vi "NI_9219_Config.vi"(8 "error in":errorcluster, 11 "task in":refnum<k21>) -> (0 "error out":errorcluster, 3 "task out":refnum<k21>)   [LabVIEW 2022 SP3]
uses:
  <vilib>/DAQmx/create/channels.llb/DAQmx Create Channel (AI-Voltage-Basic).vi
  <vilib>/DAQmx/create/channels.llb/DAQmx Create Channel (AI-Current-Basic).vi
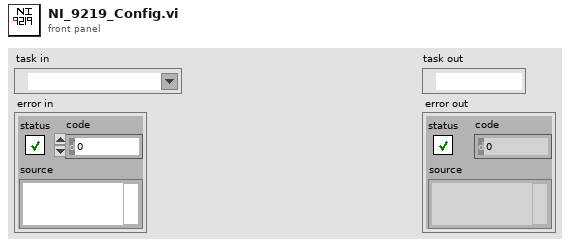
[diagram p1: front panel]
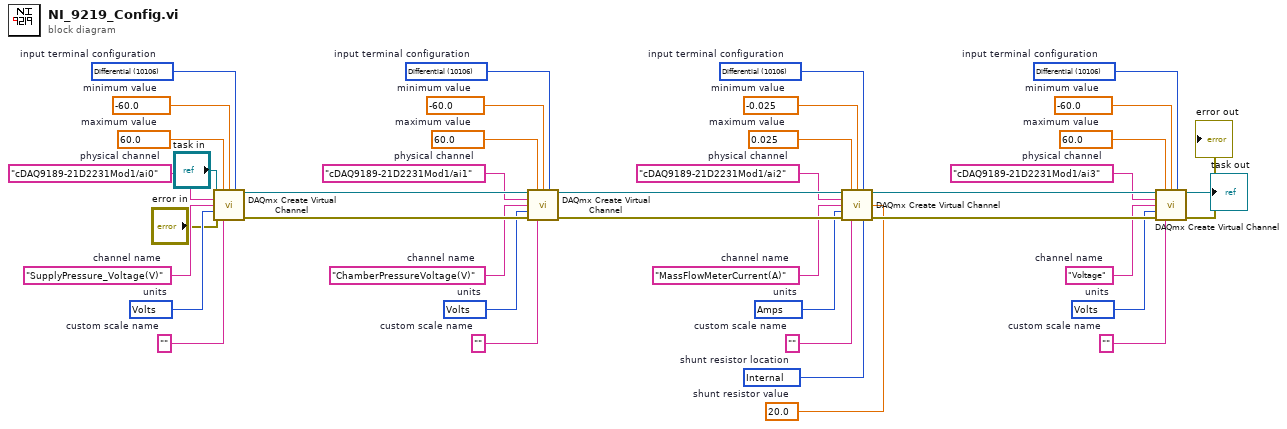
[diagram p0: block diagram]
diagram:
  w5 = 10106 items=["default"=-1, "RSE"=10083, "NRSE"=10078, "Differential"=10106, "Pseudodifferential"=12529]  # input terminal configuration
  w6 = 10348 items=["Volts"=10348, "From Custom Scale"=10065]  # units
  w7 = "Voltage"  # channel name
  w8 = ""  # custom scale name
  w9 = -60.0  # minimum value
  w10 = 60.0  # maximum value
  w11 = "cDAQ9189-21D2231Mod1/ai3"  # physical channel
  w13 = 10106 items=["default"=-1, "RSE"=10083, "NRSE"=10078, "Differential"=10106, "Pseudodifferential"=12529]  # input terminal configuration
  w14 = 10342 items=["Amps"=10342, "From Custom Scale"=10065]  # units
  w15 = 20.0  # shunt resistor value
  w16 = 10200 items=["Internal"=10200, "External"=10167]  # shunt resistor location
  w17 = "MassFlowMeterCurrent(A)"  # channel name
  w19 = ""  # custom scale name
  w20 = -0.025  # minimum value
  w21 = 0.025  # maximum value
  w22 = "cDAQ9189-21D2231Mod1/ai2"  # physical channel
  w24 = 10106 items=["default"=-1, "RSE"=10083, "NRSE"=10078, "Differential"=10106, "Pseudodifferential"=12529]  # input terminal configuration
  w25 = 10348 items=["Volts"=10348, "From Custom Scale"=10065]  # units
  w26 = "ChamberPressureVoltage(V)"  # channel name
  w28 = ""  # custom scale name
  w29 = -60.0  # minimum value
  w30 = 60.0  # maximum value
  w31 = "cDAQ9189-21D2231Mod1/ai1"  # physical channel
  w33 = 10106 items=["default"=-1, "RSE"=10083, "NRSE"=10078, "Differential"=10106, "Pseudodifferential"=12529]  # input terminal configuration
  w34 = 10348 items=["Volts"=10348, "From Custom Scale"=10065]  # units
  w35 = "SupplyPressure_Voltage(V)"  # channel name
  w37 = ""  # custom scale name
  w38 = -60.0  # minimum value
  w39 = 60.0  # maximum value
  w40 = "cDAQ9189-21D2231Mod1/ai0"  # physical channel
  n1 = call-poly <vilib>:"DAQmx Create Virtual Channel.vi"("task in"="task in", "maximum value"=w39, "minimum value"=w38, "input terminal configuration"=w33, "physical channels"=w40, "name to assign"=w35, "units"=w34, "error in"="error in", "custom scale name"=w37) -> ("task out"=w32:refnum<k21>, "error out"=w36:errorcluster)  [unwired: 5 in]
  n2 = call-poly <vilib>:"DAQmx Create Virtual Channel.vi"("task in"=w32, "maximum value"=w30, "minimum value"=w29, "input terminal configuration"=w24, "physical channels"=w31, "name to assign"=w26, "units"=w25, "error in"=w36, "custom scale name"=w28) -> ("task out"=w23:refnum<k21>, "error out"=w27:errorcluster)  [unwired: 5 in]
  n3 = call-poly <vilib>:"DAQmx Create Virtual Channel.vi"("task in"=w23, "maximum value"=w21, "minimum value"=w20, "input terminal configuration"=w13, "physical channels"=w22, "name to assign"=w17, "external shunt resistor value"=w15, "units"=w14, "error in"=w27, "custom scale name"=w19, "shunt resistor location"=w16) -> ("task out"=w12:refnum<k21>, "error out"=w18:errorcluster)  [unwired: 3 in]
  n4 = call-poly <vilib>:"DAQmx Create Virtual Channel.vi"("task in"=w12, "maximum value"=w10, "minimum value"=w9, "input terminal configuration"=w5, "physical channels"=w11, "name to assign"=w7, "units"=w6, "error in"=w18, "custom scale name"=w8) -> ("task out"=→"task out":refnum<k21>, "error out"=→"error out":errorcluster)  [unwired: 5 in]
